vi "Response String.vi"(8 "error in (no error)":errorcluster, 11 "ProtobufResponse in":refnum<class "ProtobufResponse.lvclass">) -> (0 "error out":errorcluster, 2 "Response String":string, 3 "ProtobufResponse out":refnum<class "ProtobufResponse.lvclass">)   [LabVIEW 2020, in "Vecto.lvlib" / "ProtobufResponse.lvclass"]
uses:
  ProtobufResponse.lvclass
  C:/Program Files (x86)/National Instruments/LabVIEW 2024/vi.lib/IlluminatedG/IG HTTP Utils/HTTP Utils/Response/Response.lvclass
  ProtobufResponse.lvclass/ProtobufResponse.ctl
  <vilib>/IlluminatedG/IG Protoc/LV-Proto/Message/Message.lvclass
  <vilib>/IlluminatedG/IG HTTP Utils/HTTP Utils/Response/Response.lvclass
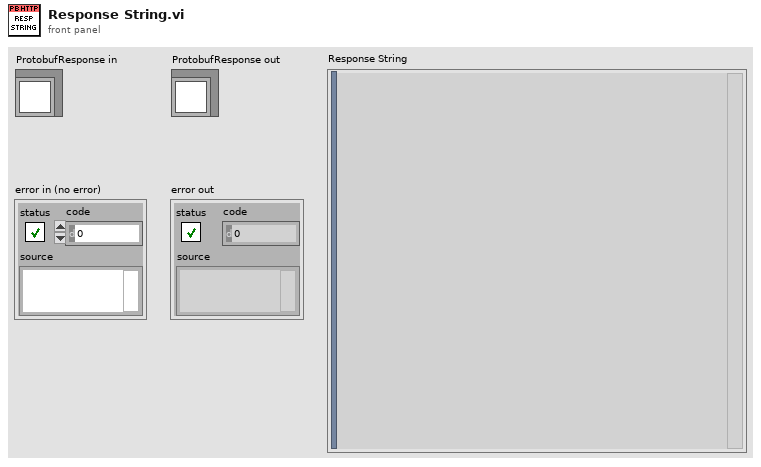
[diagram p1: front panel]
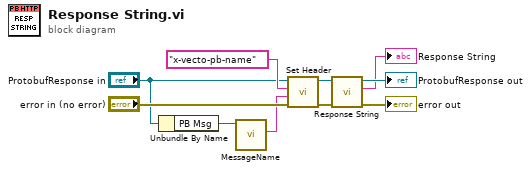
[diagram p0: block diagram]
diagram:
  n1 = Unbundle By Name("ProtobufResponse in") -> ("PB Msg"=w3:refnum<class "Message.lvclass">)
  n2 = call-dynamic "MessageName.vi"("Message in"=w3) -> ("MessageName"=w2:string)  [unwired: 10 in]
  n3 = call <vilib>:"Set Header.vi"("error in (no error)"="error in (no error)", "Value"=w2, "Header"="x-vecto-pb-name", "Response in"="ProtobufResponse in") -> ("error out"=w7:errorcluster, "Response out"=w6:refnum<class "ProtobufResponse.lvclass">)  [unwired: 5 in, 1 out]
  n4 = call-parent "Response String.vi"("error in (no error)"=w7, "Response in"=w6) -> ("error out"=→"error out":errorcluster, "Response String"=→"Response String":string, "Response out"=→"ProtobufResponse out":refnum<class "ProtobufResponse.lvclass">)  [unwired: 7 in]
